vi "Initialize.vi"(8 "error in (no error)":errorcluster, 9 "reset (T:yes)":bool=TRUE, 11 "VISA resource name":refnum<visa-resource-name>) -> (0 "error out":errorcluster, 3 "VISA resource name out":refnum<visa-resource-name>)   [LabVIEW 2017, in "Fluke 8840.lvlib"]
doc: "This VI loads the addressing information about the instrument into the Open Instrument VI and returns the instrument ID. You can reset the instrument by setting the front panel reset control. You must run this VI before using any of the instrument driver VIs for this instrument."
uses:
  Fluke 8840.lvlib
panel:
  # "Copyright 2005. National Instruments Corporation."
  # "yes\nno"
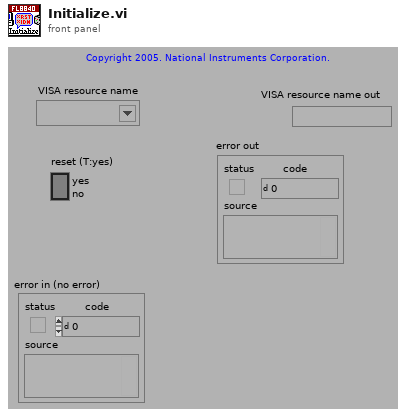
[diagram p1: front panel]
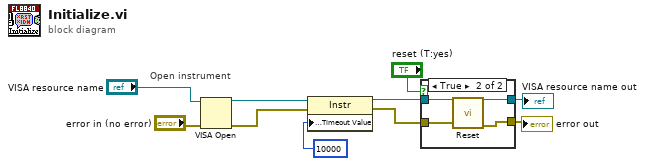
[diagram p0: block diagram]
diagram:
  # "Open instrument"
  n1 = VISA Open(error in (no error)="error in (no error)", VISA resource name="VISA resource name") -> (VISA resource name=w2:refnum<visa-resource-name>, error out=w1:errorcluster)  [unwired: 3 out]
  n2 = property class="Instr"(reference=w2, error in=w1, "General Settings:Timeout Value"=u32 10000 ("Tmo Value")) -> (reference out=w4:refnum<visa-resource-name>, error out=w3:errorcluster)
  n3 = case shown="True" "reset (T:yes)" {
    tunnel: w4 -> [w12 w16]
    tunnel: w3 -> [w11 w15]
    tunnel: [w12 w14] -> w8
    tunnel: [w11 w13] -> w7
    frame False {
    }
    frame True {
      n4 = call "Reset.vi"("error in (no error)"=w15, "VISA resource name"=w16) -> ("error out"=w13:errorcluster, "VISA resource name out"=w14:refnum<visa-resource-name>)  [unwired: 8 out]
    }
  }
  "VISA resource name out" <- w8
  "error out" <- w7
